vi "HolDrvCtrl_AdvCalculate_Trajectory.vi"(7 "currentPose":T2={"TRANSLATION"={"X"=0.0, "Y"=0.0}, "ROTATION"={"VALUE"=0.0, "COS"=1.0, "SIN"=0.0}} {"ROTATION"."SIN" format="%13.4f"; "ROTATION"."COS" format="%13.4f"; "ROTATION"."VALUE" format="%13.4f"; "TRANSLATION"."Y" format="%14.3f"; "TRANSLATION"."X" format="%14.3f"}, 8 "angleRef":T4={"VALUE"=0.0, "COS"=1.0, "SIN"=0.0} {"SIN" format="%13.4f"; "COS" format="%13.4f"; "VALUE" format="%13.4f"}, 10 "desiredTrajState":T1={"TimeSeconds"=0.0, "Velocity"=0.0, "Acceleration"=0.0, "POSE"={"TRANSLATION"={"X"=0.0, "Y"=0.0}, "ROTATION"={"VALUE"=0.0, "COS"=1.0, "SIN"=0.0}}, "Curvature"=0.0} {"POSE"."ROTATION"."SIN" format="%13.4f"; "POSE"."ROTATION"."COS" format="%13.4f"; "POSE"."ROTATION"."VALUE" format="%13.4f"; "POSE"."TRANSLATION"."Y" format="%14.3f"; "POSE"."TRANSLATION"."X" format="%14.3f"}, 11 "inHOLONOMIC_DRV_CTRL":T6={"poseTolerance"={"TRANSLATION"={"X"=0.0, "Y"=0.0}, "ROTATION"={"VALUE"=0.0, "COS"=1.0, "SIN"=0.0}}, "poseError"={"TRANSLATION"={"X"=0.0, "Y"=0.0}, "ROTATION"={"VALUE"=0.0, "COS"=1.0, "SIN"=0.0}}, "Enabled"=TRUE, "PID_xCtrl"={"Kp"=0.0, "Ki"=0.0, "Kd"=0.0, "Period"=0.0, "Max_Integral"=1.0, "Min_Integral"=-1.0, "Max_Input"=0.0, "Min_Input"=0.0, "Continuous"=FALSE, "PositionError"=0.0, "VelocityError"=0.0, "PrevError"=0.0, "TotalError"=0.0, "PositionTolerance"=0.05, "VelocityTolerance"=9.99e+35, "SetPoint"=0.0, "Kf"=0.0, "Prev_Deriv"=0.0, "Prev_Deriv 2"=0.0, "DerivativeFilter"=FALSE, "Min_Output"=-9.99e+35, "Max_Output"=9.9e+35, "Prev_F_P"=0.0, "Prev_F_P_2"=0.0, "AntiWindupActive"=FALSE, "Measurement"=0.0}, "PID_yCtrl"={"Kp"=0.0, "Ki"=0.0, "Kd"=0.0, "Period"=0.0, "Max_Integral"=1.0, "Min_Integral"=-1.0, "Max_Input"=0.0, "Min_Input"=0.0, "Continuous"=FALSE, "PositionError"=0.0, "VelocityError"=0.0, "PrevError"=0.0, "TotalError"=0.0, "PositionTolerance"=0.05, "VelocityTolerance"=9.99e+35, "SetPoint"=0.0, "Kf"=0.0, "Prev_Deriv"=0.0, "Prev_Deriv 2"=0.0, "DerivativeFilter"=FALSE, "Min_Output"=-9.99e+35, "Max_Output"=9.9e+35, "Prev_F_P"=0.0, "Prev_F_P_2"=0.0, "AntiWindupActive"=FALSE, "Measurement"=0.0}, "PROF_PID_thetaCtrl"={"Controller"={"Kp"=0.0, "Ki"=0.0, "Kd"=0.0, "Period"=0.0, "Max_Integral"=1.0, "Min_Integral"=-1.0, "Max_Input"=0.0, "Min_Input"=0.0, "Continuous"=FALSE, "PositionError"=0.0, "VelocityError"=0.0, "PrevError"=0.0, "TotalError"=0.0, "PositionTolerance"=0.05, "VelocityTolerance"=9.99e+35, "SetPoint"=0.0, "Kf"=0.0, "Prev_Deriv"=0.0, "Prev_Deriv 2"=0.0, "DerivativeFilter"=FALSE, "Min_Output"=-9.99e+35, "Max_Output"=9.9e+35, "Prev_F_P"=0.0, "Prev_F_P_2"=0.0, "AntiWindupActive"=FALSE, "Measurement"=0.0}, "Goal"={"Position"=0.0, "Velocity"=0.0}, "Setpoint"={"Position"=0.0, "Velocity"=0.0}, "Constraint"={"MaxVelocity"=0.0, "MaxAcceleration"=0.0}}, "RotationError"={"VALUE"=0.0, "COS"=1.0, "SIN"=0.0}, "FirstRun"=TRUE} {"RotationError"."SIN" format="%13.4f"; "RotationError"."COS" format="%13.4f"; "RotationError"."VALUE" format="%13.4f"; "PROF_PID_thetaCtrl"."Constraint"."MaxAcceleration" format="%16_6e"; "PROF_PID_thetaCtrl"."Constraint"."MaxVelocity" format="%16_6e"; "PROF_PID_thetaCtrl"."Setpoint"."Velocity" format="%16_6e"; "PROF_PID_thetaCtrl"."Setpoint"."Position" format="%16_6e"; "PROF_PID_thetaCtrl"."Goal"."Velocity" format="%16_6e"; "PROF_PID_thetaCtrl"."Goal"."Position" format="%16_6e"; "PROF_PID_thetaCtrl"."Controller"."Measurement" format="%16_6e"; "PROF_PID_thetaCtrl"."Controller"."Prev_F_P_2" format="%16_6e"; "PROF_PID_thetaCtrl"."Controller"."Prev_F_P" format="%16_6e"; "PROF_PID_thetaCtrl"."Controller"."Max_Output" format="%16_6e"; "PROF_PID_thetaCtrl"."Controller"."Min_Output" format="%16_6e"; "PROF_PID_thetaCtrl"."Controller"."Prev_Deriv 2" format="%16_6e"; "PROF_PID_thetaCtrl"."Controller"."Prev_Deriv" format="%16_6e"; "PROF_PID_thetaCtrl"."Controller"."Kf" format="%16_6e"; "PROF_PID_thetaCtrl"."Controller"."SetPoint" format="%16_6e"; "PROF_PID_thetaCtrl"."Controller"."VelocityTolerance" format="%16_6e"; "PROF_PID_thetaCtrl"."Controller"."PositionTolerance" format="%16_6e"; "PROF_PID_thetaCtrl"."Controller"."TotalError" format="%16_6e"; "PROF_PID_thetaCtrl"."Controller"."PrevError" format="%16_6e"; "PROF_PID_thetaCtrl"."Controller"."VelocityError" format="%16_6e"; "PROF_PID_thetaCtrl"."Controller"."PositionError" format="%16_6e"; "PROF_PID_thetaCtrl"."Controller"."Min_Input" format="%16_6e"; "PROF_PID_thetaCtrl"."Controller"."Max_Input" format="%16_6e"; "PROF_PID_thetaCtrl"."Controller"."Min_Integral" format="%16_6e"; "PROF_PID_thetaCtrl"."Controller"."Max_Integral" format="%16_6e"; "PROF_PID_thetaCtrl"."Controller"."Period" format="%16_6e"; "PROF_PID_thetaCtrl"."Controller"."Kd" format="%16_6e"; "PROF_PID_thetaCtrl"."Controller"."Ki" format="%16_6e"; "PROF_PID_thetaCtrl"."Controller"."Kp" format="%16_6e"; "PID_yCtrl"."Measurement" format="%16_6e"; "PID_yCtrl"."Prev_F_P_2" format="%16_6e"; "PID_yCtrl"."Prev_F_P" format="%16_6e"; "PID_yCtrl"."Max_Output" format="%16_6e"; "PID_yCtrl"."Min_Output" format="%16_6e"; "PID_yCtrl"."Prev_Deriv 2" format="%16_6e"; "PID_yCtrl"."Prev_Deriv" format="%16_6e"; "PID_yCtrl"."Kf" format="%16_6e"; "PID_yCtrl"."SetPoint" format="%16_6e"; "PID_yCtrl"."VelocityTolerance" format="%16_6e"; "PID_yCtrl"."PositionTolerance" format="%16_6e"; "PID_yCtrl"."TotalError" format="%16_6e"; "PID_yCtrl"."PrevError" format="%16_6e"; "PID_yCtrl"."VelocityError" format="%16_6e"; "PID_yCtrl"."PositionError" format="%16_6e"; "PID_yCtrl"."Min_Input" format="%16_6e"; "PID_yCtrl"."Max_Input" format="%16_6e"; "PID_yCtrl"."Min_Integral" format="%16_6e"; "PID_yCtrl"."Max_Integral" format="%16_6e"; "PID_yCtrl"."Period" format="%16_6e"; "PID_yCtrl"."Kd" format="%16_6e"; "PID_yCtrl"."Ki" format="%16_6e"; "PID_yCtrl"."Kp" format="%16_6e"; "PID_xCtrl"."Measurement" format="%16_6e"; "PID_xCtrl"."Prev_F_P_2" format="%16_6e"; "PID_xCtrl"."Prev_F_P" format="%16_6e"; "PID_xCtrl"."Max_Output" format="%16_6e"; "PID_xCtrl"."Min_Output" format="%16_6e"; "PID_xCtrl"."Prev_Deriv 2" format="%16_6e"; "PID_xCtrl"."Prev_Deriv" format="%16_6e"; "PID_xCtrl"."Kf" format="%16_6e"; "PID_xCtrl"."SetPoint" format="%16_6e"; "PID_xCtrl"."VelocityTolerance" format="%16_6e"; "PID_xCtrl"."PositionTolerance" format="%16_6e"; "PID_xCtrl"."TotalError" format="%16_6e"; "PID_xCtrl"."PrevError" format="%16_6e"; "PID_xCtrl"."VelocityError" format="%16_6e"; "PID_xCtrl"."PositionError" format="%16_6e"; "PID_xCtrl"."Min_Input" format="%16_6e"; "PID_xCtrl"."Max_Input" format="%16_6e"; "PID_xCtrl"."Min_Integral" format="%16_6e"; "PID_xCtrl"."Max_Integral" format="%16_6e"; "PID_xCtrl"."Period" format="%16_6e"; "PID_xCtrl"."Kd" format="%16_6e"; "PID_xCtrl"."Ki" format="%16_6e"; "PID_xCtrl"."Kp" format="%16_6e"; "poseError"."ROTATION"."SIN" format="%13.4f"; "poseError"."ROTATION"."COS" format="%13.4f"; "poseError"."ROTATION"."VALUE" format="%13.4f"; "poseError"."TRANSLATION"."Y" format="%14.3f"; "poseError"."TRANSLATION"."X" format="%14.3f"; "poseTolerance"."ROTATION"."SIN" format="%13.4f"; "poseTolerance"."ROTATION"."COS" format="%13.4f"; "poseTolerance"."ROTATION"."VALUE" format="%13.4f"; "poseTolerance"."TRANSLATION"."Y" format="%14.3f"; "poseTolerance"."TRANSLATION"."X" format="%14.3f"}) -> (1 "calcChassisSpeed":T5 {"vOmega" format="%10.3f"; "vY" format="%10.3f"; "vX" format="%10.3f"}, 3 "outHOLONOMIC_DRV_CTRL":T6={"poseTolerance"={"TRANSLATION"={"X"=0.0, "Y"=0.0}, "ROTATION"={"VALUE"=0.0, "COS"=1.0, "SIN"=0.0}}, "poseError"={"TRANSLATION"={"X"=0.0, "Y"=0.0}, "ROTATION"={"VALUE"=0.0, "COS"=1.0, "SIN"=0.0}}, "Enabled"=TRUE, "PID_xCtrl"={"Kp"=0.0, "Ki"=0.0, "Kd"=0.0, "Period"=0.0, "Max_Integral"=1.0, "Min_Integral"=-1.0, "Max_Input"=0.0, "Min_Input"=0.0, "Continuous"=FALSE, "PositionError"=0.0, "VelocityError"=0.0, "PrevError"=0.0, "TotalError"=0.0, "PositionTolerance"=0.05, "VelocityTolerance"=9.99e+35, "SetPoint"=0.0, "Kf"=0.0, "Prev_Deriv"=0.0, "Prev_Deriv 2"=0.0, "DerivativeFilter"=FALSE, "Min_Output"=-9.99e+35, "Max_Output"=9.9e+35, "Prev_F_P"=0.0, "Prev_F_P_2"=0.0, "AntiWindupActive"=FALSE, "Measurement"=0.0}, "PID_yCtrl"={"Kp"=0.0, "Ki"=0.0, "Kd"=0.0, "Period"=0.0, "Max_Integral"=1.0, "Min_Integral"=-1.0, "Max_Input"=0.0, "Min_Input"=0.0, "Continuous"=FALSE, "PositionError"=0.0, "VelocityError"=0.0, "PrevError"=0.0, "TotalError"=0.0, "PositionTolerance"=0.05, "VelocityTolerance"=9.99e+35, "SetPoint"=0.0, "Kf"=0.0, "Prev_Deriv"=0.0, "Prev_Deriv 2"=0.0, "DerivativeFilter"=FALSE, "Min_Output"=-9.99e+35, "Max_Output"=9.9e+35, "Prev_F_P"=0.0, "Prev_F_P_2"=0.0, "AntiWindupActive"=FALSE, "Measurement"=0.0}, "PROF_PID_thetaCtrl"={"Controller"={"Kp"=0.0, "Ki"=0.0, "Kd"=0.0, "Period"=0.0, "Max_Integral"=1.0, "Min_Integral"=-1.0, "Max_Input"=0.0, "Min_Input"=0.0, "Continuous"=FALSE, "PositionError"=0.0, "VelocityError"=0.0, "PrevError"=0.0, "TotalError"=0.0, "PositionTolerance"=0.05, "VelocityTolerance"=9.99e+35, "SetPoint"=0.0, "Kf"=0.0, "Prev_Deriv"=0.0, "Prev_Deriv 2"=0.0, "DerivativeFilter"=FALSE, "Min_Output"=-9.99e+35, "Max_Output"=9.9e+35, "Prev_F_P"=0.0, "Prev_F_P_2"=0.0, "AntiWindupActive"=FALSE, "Measurement"=0.0}, "Goal"={"Position"=0.0, "Velocity"=0.0}, "Setpoint"={"Position"=0.0, "Velocity"=0.0}, "Constraint"={"MaxVelocity"=0.0, "MaxAcceleration"=0.0}}, "RotationError"={"VALUE"=0.0, "COS"=1.0, "SIN"=0.0}, "FirstRun"=TRUE} {"RotationError"."SIN" format="%13.4f"; "RotationError"."COS" format="%13.4f"; "RotationError"."VALUE" format="%13.4f"; "PROF_PID_thetaCtrl"."Constraint"."MaxAcceleration" format="%16_6e"; "PROF_PID_thetaCtrl"."Constraint"."MaxVelocity" format="%16_6e"; "PROF_PID_thetaCtrl"."Setpoint"."Velocity" format="%16_6e"; "PROF_PID_thetaCtrl"."Setpoint"."Position" format="%16_6e"; "PROF_PID_thetaCtrl"."Goal"."Velocity" format="%16_6e"; "PROF_PID_thetaCtrl"."Goal"."Position" format="%16_6e"; "PROF_PID_thetaCtrl"."Controller"."Measurement" format="%16_6e"; "PROF_PID_thetaCtrl"."Controller"."Prev_F_P_2" format="%16_6e"; "PROF_PID_thetaCtrl"."Controller"."Prev_F_P" format="%16_6e"; "PROF_PID_thetaCtrl"."Controller"."Max_Output" format="%16_6e"; "PROF_PID_thetaCtrl"."Controller"."Min_Output" format="%16_6e"; "PROF_PID_thetaCtrl"."Controller"."Prev_Deriv 2" format="%16_6e"; "PROF_PID_thetaCtrl"."Controller"."Prev_Deriv" format="%16_6e"; "PROF_PID_thetaCtrl"."Controller"."Kf" format="%16_6e"; "PROF_PID_thetaCtrl"."Controller"."SetPoint" format="%16_6e"; "PROF_PID_thetaCtrl"."Controller"."VelocityTolerance" format="%16_6e"; "PROF_PID_thetaCtrl"."Controller"."PositionTolerance" format="%16_6e"; "PROF_PID_thetaCtrl"."Controller"."TotalError" format="%16_6e"; "PROF_PID_thetaCtrl"."Controller"."PrevError" format="%16_6e"; "PROF_PID_thetaCtrl"."Controller"."VelocityError" format="%16_6e"; "PROF_PID_thetaCtrl"."Controller"."PositionError" format="%16_6e"; "PROF_PID_thetaCtrl"."Controller"."Min_Input" format="%16_6e"; "PROF_PID_thetaCtrl"."Controller"."Max_Input" format="%16_6e"; "PROF_PID_thetaCtrl"."Controller"."Min_Integral" format="%16_6e"; "PROF_PID_thetaCtrl"."Controller"."Max_Integral" format="%16_6e"; "PROF_PID_thetaCtrl"."Controller"."Period" format="%16_6e"; "PROF_PID_thetaCtrl"."Controller"."Kd" format="%16_6e"; "PROF_PID_thetaCtrl"."Controller"."Ki" format="%16_6e"; "PROF_PID_thetaCtrl"."Controller"."Kp" format="%16_6e"; "PID_yCtrl"."Measurement" format="%16_6e"; "PID_yCtrl"."Prev_F_P_2" format="%16_6e"; "PID_yCtrl"."Prev_F_P" format="%16_6e"; "PID_yCtrl"."Max_Output" format="%16_6e"; "PID_yCtrl"."Min_Output" format="%16_6e"; "PID_yCtrl"."Prev_Deriv 2" format="%16_6e"; "PID_yCtrl"."Prev_Deriv" format="%16_6e"; "PID_yCtrl"."Kf" format="%16_6e"; "PID_yCtrl"."SetPoint" format="%16_6e"; "PID_yCtrl"."VelocityTolerance" format="%16_6e"; "PID_yCtrl"."PositionTolerance" format="%16_6e"; "PID_yCtrl"."TotalError" format="%16_6e"; "PID_yCtrl"."PrevError" format="%16_6e"; "PID_yCtrl"."VelocityError" format="%16_6e"; "PID_yCtrl"."PositionError" format="%16_6e"; "PID_yCtrl"."Min_Input" format="%16_6e"; "PID_yCtrl"."Max_Input" format="%16_6e"; "PID_yCtrl"."Min_Integral" format="%16_6e"; "PID_yCtrl"."Max_Integral" format="%16_6e"; "PID_yCtrl"."Period" format="%16_6e"; "PID_yCtrl"."Kd" format="%16_6e"; "PID_yCtrl"."Ki" format="%16_6e"; "PID_yCtrl"."Kp" format="%16_6e"; "PID_xCtrl"."Measurement" format="%16_6e"; "PID_xCtrl"."Prev_F_P_2" format="%16_6e"; "PID_xCtrl"."Prev_F_P" format="%16_6e"; "PID_xCtrl"."Max_Output" format="%16_6e"; "PID_xCtrl"."Min_Output" format="%16_6e"; "PID_xCtrl"."Prev_Deriv 2" format="%16_6e"; "PID_xCtrl"."Prev_Deriv" format="%16_6e"; "PID_xCtrl"."Kf" format="%16_6e"; "PID_xCtrl"."SetPoint" format="%16_6e"; "PID_xCtrl"."VelocityTolerance" format="%16_6e"; "PID_xCtrl"."PositionTolerance" format="%16_6e"; "PID_xCtrl"."TotalError" format="%16_6e"; "PID_xCtrl"."PrevError" format="%16_6e"; "PID_xCtrl"."VelocityError" format="%16_6e"; "PID_xCtrl"."PositionError" format="%16_6e"; "PID_xCtrl"."Min_Input" format="%16_6e"; "PID_xCtrl"."Max_Input" format="%16_6e"; "PID_xCtrl"."Min_Integral" format="%16_6e"; "PID_xCtrl"."Max_Integral" format="%16_6e"; "PID_xCtrl"."Period" format="%16_6e"; "PID_xCtrl"."Kd" format="%16_6e"; "PID_xCtrl"."Ki" format="%16_6e"; "PID_xCtrl"."Kp" format="%16_6e"; "poseError"."ROTATION"."SIN" format="%13.4f"; "poseError"."ROTATION"."COS" format="%13.4f"; "poseError"."ROTATION"."VALUE" format="%13.4f"; "poseError"."TRANSLATION"."Y" format="%14.3f"; "poseError"."TRANSLATION"."X" format="%14.3f"; "poseTolerance"."ROTATION"."SIN" format="%13.4f"; "poseTolerance"."ROTATION"."COS" format="%13.4f"; "poseTolerance"."ROTATION"."VALUE" format="%13.4f"; "poseTolerance"."TRANSLATION"."Y" format="%14.3f"; "poseTolerance"."TRANSLATION"."X" format="%14.3f"})   [LabVIEW 2019, in "Trajectory_Library.lvlib"]
doc: "Returns the next output of the holonomic drive controller.\n\nThis version uses the Advanced PID instead of the standard PID for X and Y control.\n\nInputs:\n - inHolonomicDrvCtrl -- controller data structure\n - currentPose -- The current pose.\n - desiredState -- The desired trajectory state.\n - angleRef -- The desired end-angle.\n\nOutputs:\n - outHolonomicDrvCtrl -- updated controller data structure\n - calcChassisSpeed -- The next output of the holonomic drive controller."
uses:
  Trajectory_Library.lvlib
  HOLONOMIC_DRV_CTRL.ctl
  POSE2D.ctl
  TRANSLATION2D.ctl
  ROTATION2D.ctl
  PID_CONTROLLER.ctl
  PROFILED_PID_CONTROLLER.ctl
  TRAPEZOID_PROFILE_STATE.ctl
  TRAPEZOID_PROFILE_CONSTRAINT.ctl
  CHASSIS_SPEEDS.ctl
  TRAJ_STATE.ctl
  ProfiledPIDController_Calculate_Meas_Goal.vi
  ProfiledPIDController_Reset_PosOnly.vi
  ChassisSpeeds_FromFieldRelativeSpeeds.vi
  Pose_getXYAngle.vi
  Rotation_GetAngleCosSin.vi
  Pose_RelativeTo.vi
  Pose_getRotation.vi
  Rotation_Minus.vi
  ProfiledPIDController_SetGoal_PosOnly.vi
  ProfiledPIDController_Calculate_Meas.vi
  TrapProfState_New.vi
  ProfiledPIDController_Reset.vi
  Rotation_GetCos.vi
  Rotation_GetSin.vi
  ChassisSpeeds_New.vi
  Transform_Create_PosePose.vi
  Pose_New_TRRO.vi
  Rotation_UnaryMinus.vi
  Rotation_RotateBy.vi
  ProfiledPIDController_SetGoal.vi
  PIDController_Calculate_SP_PV.vi
  TrapProfile_New.vi
  ProfiledPIDController_GetPeriod.vi
  TrapProfile_Calculate.vi
  ControllerUtil_GetModulusError.vi
  PIDController_Reset.vi
  Translation_RotateBy.vi
  Translation_Minus.vi
  Rotation_CreateAngle.vi
  Rotation_CreateXY.vi
  PIDController_SetSetpoint.vi
  PIDController_Calculate_PV.vi
  TrapProfile_ShouldFlipAcceleration.vi
  TrapProfile_Direct.vi
  <vilib>/Rock Robotics/SystemInterfaces/NetworkCommunication/NetComm_UsageReport_report.vi
  PIDController_GetPeriod.vi
  Translation_Create.vi
  Util_CalcDist.vi
  PIDController_AdvCalculate_FF_Sp_Pv.vi
  Util_LibraryGlobals.vi
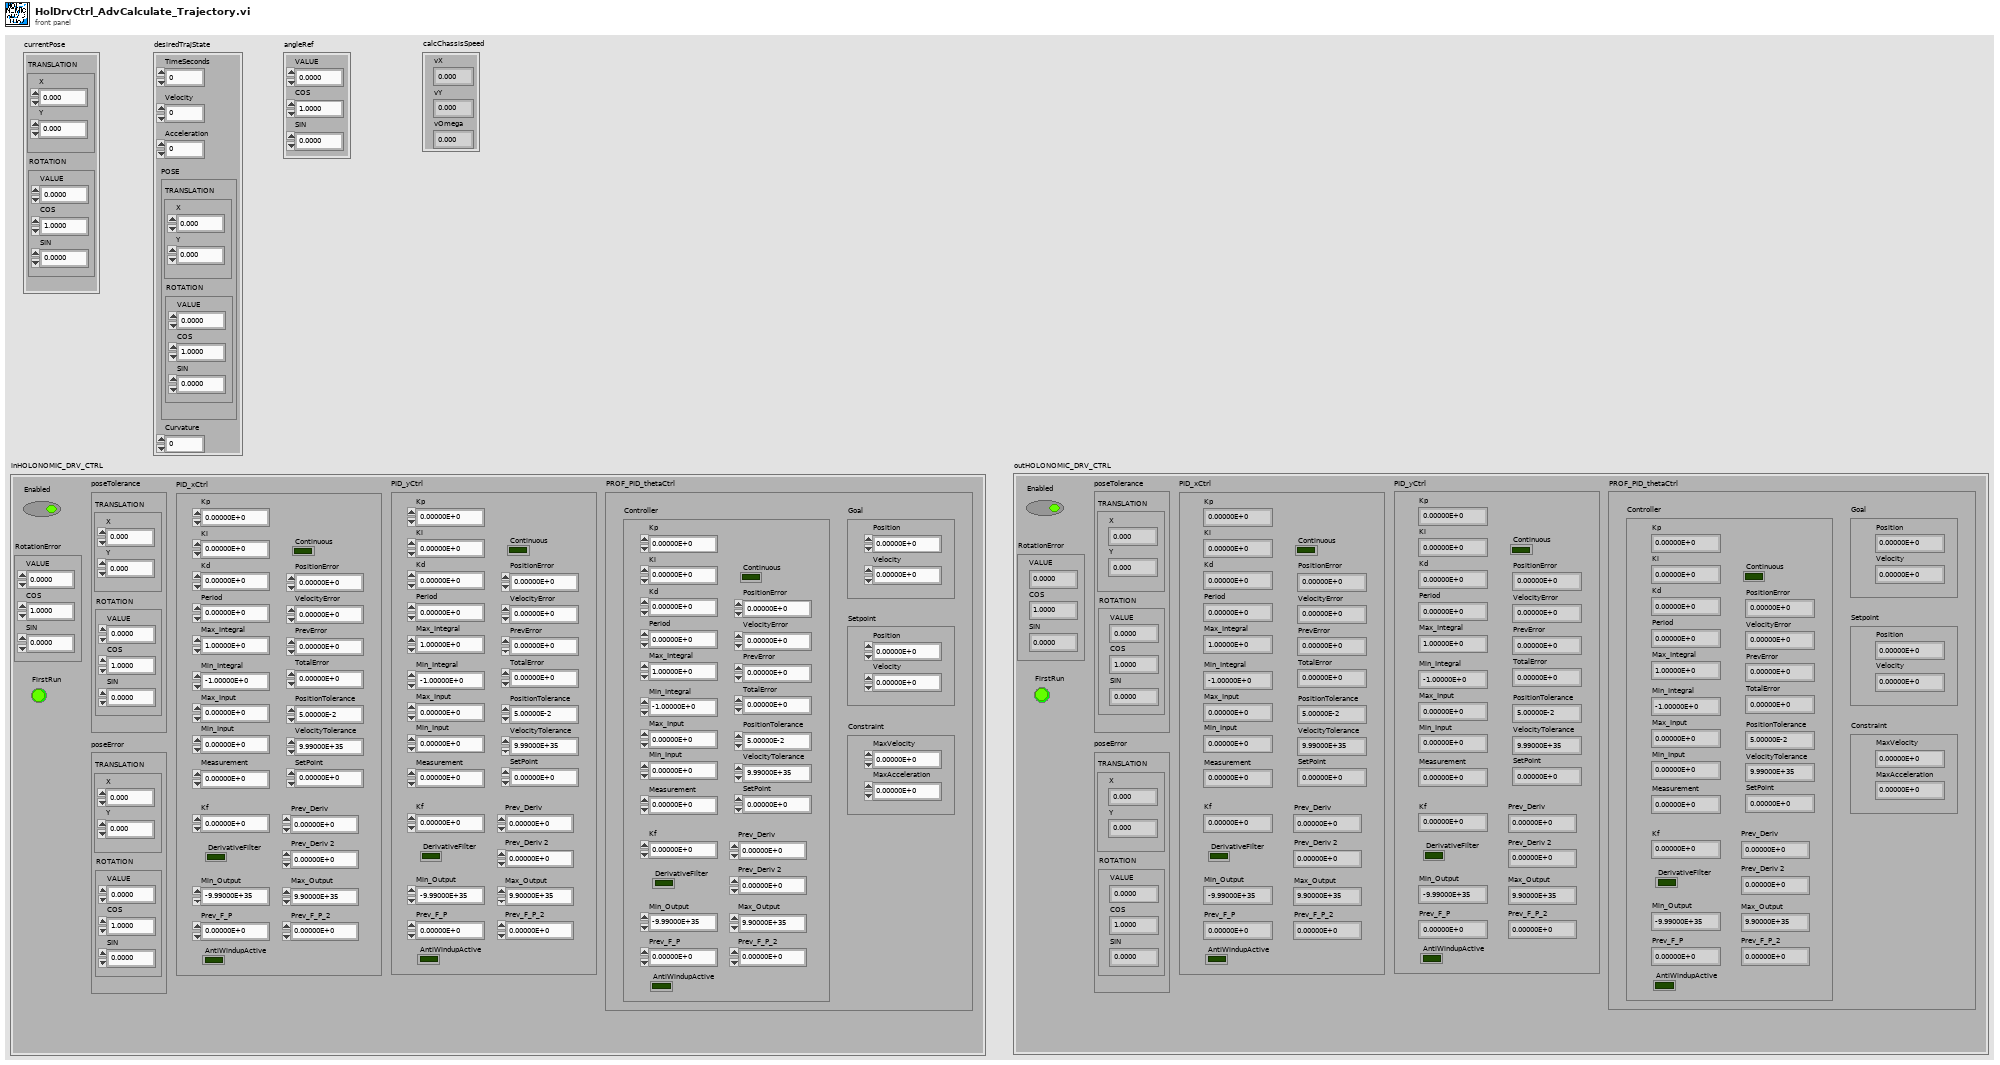
[diagram p1: front panel]
types:
  T1 = typedef "Trajectory_Library.lvlib/TRAJ_STATE.ctl" = cluster{"TimeSeconds":dbl, "Velocity":dbl, "Acceleration":dbl, "POSE":T2, "Curvature":dbl}
  T2 = typedef "Trajectory_Library.lvlib/POSE2D.ctl" = cluster{"TRANSLATION":T3, "ROTATION":T4}
  T3 = typedef "Trajectory_Library.lvlib/TRANSLATION2D.ctl" = cluster{"X":dbl, "Y":dbl}
  T4 = typedef "Trajectory_Library.lvlib/ROTATION2D.ctl" = cluster{"VALUE":dbl, "COS":dbl, "SIN":dbl}
  T5 = typedef "Trajectory_Library.lvlib/CHASSIS_SPEEDS.ctl" = cluster{"vX":dbl, "vY":dbl, "vOmega":dbl}
  T6 = typedef "Trajectory_Library.lvlib/HOLONOMIC_DRV_CTRL.ctl" = cluster{"poseTolerance":T2, "poseError":T2, "Enabled":bool, "PID_xCtrl":T7, "PID_yCtrl":T7, "PROF_PID_thetaCtrl":T8, "RotationError":T4, "FirstRun":bool}
  T7 = typedef "Trajectory_Library.lvlib/PID_CONTROLLER.ctl" = cluster{"Kp":dbl, "Ki":dbl, "Kd":dbl, "Period":dbl, "Max_Integral":dbl, "Min_Integral":dbl, "Max_Input":dbl, "Min_Input":dbl, "Continuous":bool, "PositionError":dbl, "VelocityError":dbl, "PrevError":dbl, "TotalError":dbl, "PositionTolerance":dbl, "VelocityTolerance":dbl, "SetPoint":dbl, "Kf":dbl, "Prev_Deriv":dbl, "Prev_Deriv 2":dbl, "DerivativeFilter":bool, "Min_Output":dbl, "Max_Output":dbl, "Prev_F_P":dbl, "Prev_F_P_2":dbl, "AntiWindupActive":bool, "Measurement":dbl}
  T8 = typedef "Trajectory_Library.lvlib/PROFILED_PID_CONTROLLER.ctl" = cluster{"Controller":T7, "Goal":T9, "Setpoint":T9, "Constraint":T10}
  T9 = typedef "Trajectory_Library.lvlib/TRAPEZOID_PROFILE_STATE.ctl" = cluster{"Position":dbl, "Velocity":dbl}
  T10 = typedef "Trajectory_Library.lvlib/TRAPEZOID_PROFILE_CONSTRAINT.ctl" = cluster{"MaxVelocity":dbl, "MaxAcceleration":dbl}
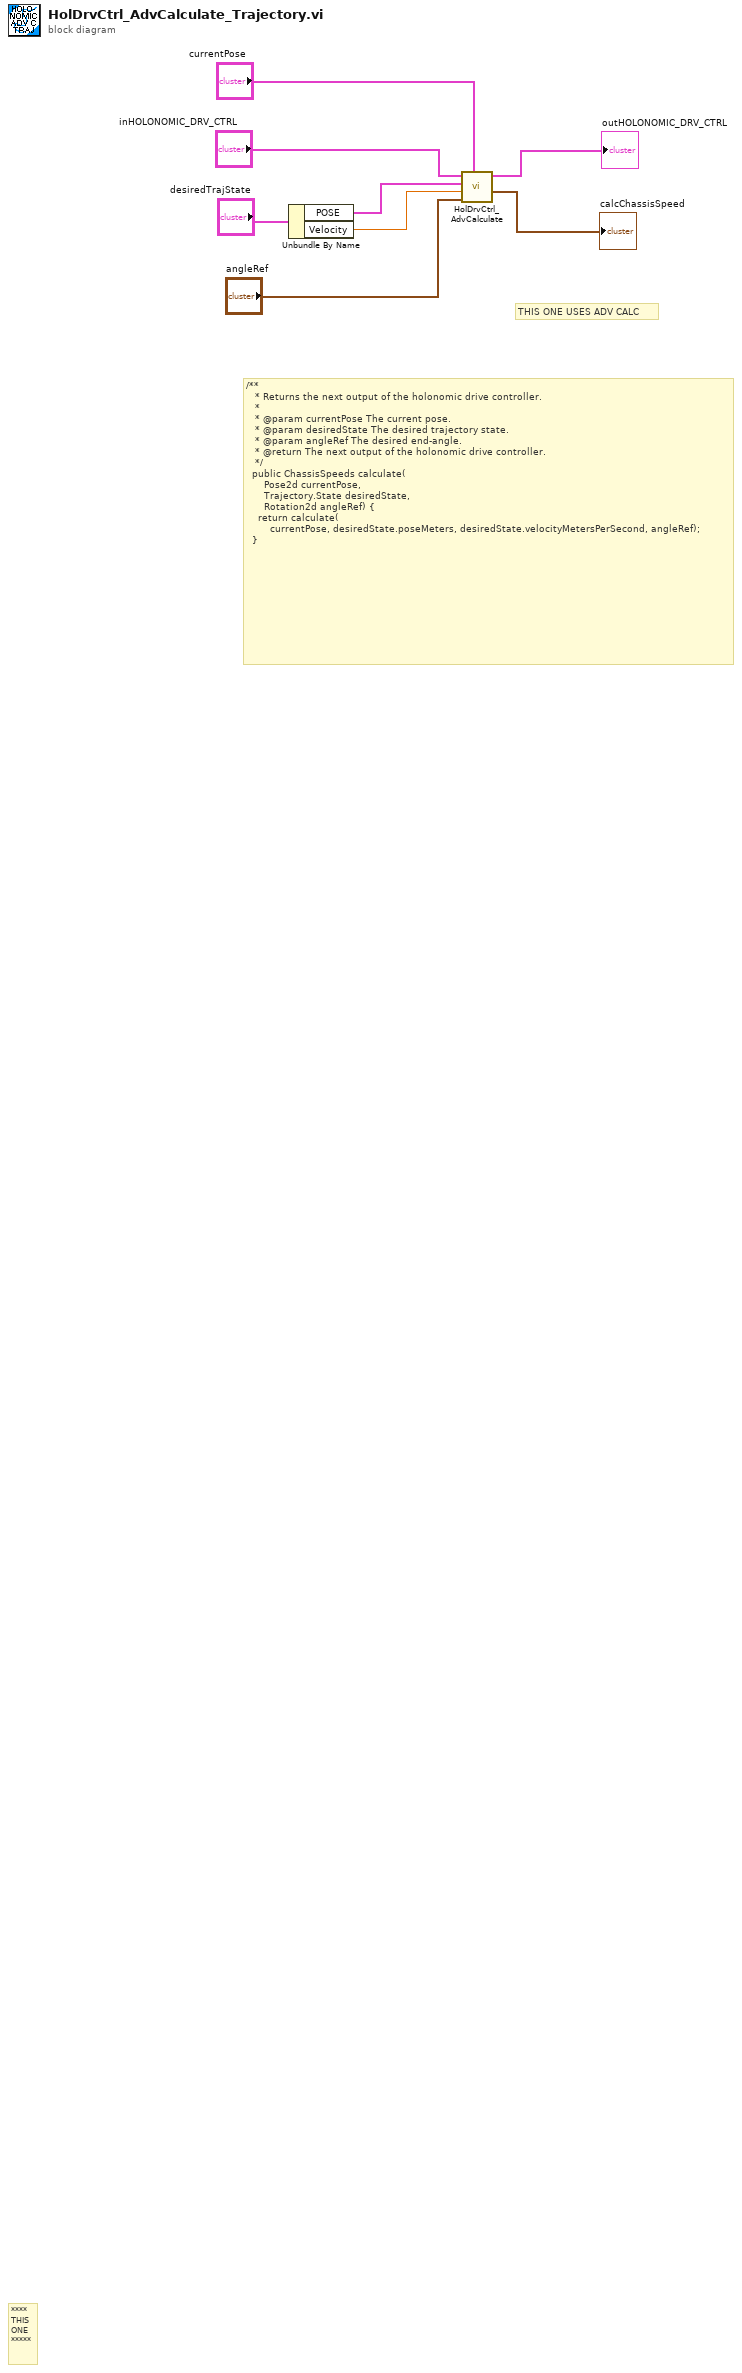
[diagram p0: block diagram]
diagram:
  # "THIS ONE USES ADV CALC"
  # "****\nTHIS\nONE\n*****"
  # "/**\n   * Returns the next output of the holonomic drive controller.\n   *\n   * @param currentPose The current pose.\n   * @param desiredState The desired trajectory state.\n   * @param angleRef The desired end-angle.\n   * @return The next output of the holonomic drive controller.\n   */\n  public ChassisSpeeds calculate(\n      Pose2d currentPose, \n      Trajectory.State desiredState, \n      Rotation2d angleRef) {\n    return calculate(\n        currentPose, desiredState.poseMeters, desiredState.velocityMetersPerSecond, angleRef);\n  }"
  n1 = Unbundle By Name("desiredTrajState") -> ("POSE"=w2:T2, "Velocity"=w1:dbl)
  n2 = call "HolDrvCtrl_AdvCalculate.vi"("currentPose"="currentPose", "angleRef"="angleRef", "linearVelRef"=w1, "poseRef"=w2, "inHOLONOMIC_DRV_CTRL"="inHOLONOMIC_DRV_CTRL") -> ("calcChassisSpeed"=→"calcChassisSpeed":T5, "outHOLONOMIC_DRV_CTRL"=→"outHOLONOMIC_DRV_CTRL":T6)  [unwired: 5 in]
